vi "Write Setpoint.vi"(8 "error in (no error)":errorcluster, 10 "Setpoint":dbl=1.0, 11 "Percent Difference in":refnum<class "Percent Difference.lvclass">) -> (0 "error out":errorcluster, 3 "Percent Difference out":refnum<class "Percent Difference.lvclass">)   [LabVIEW 2021, in "Percent Difference.lvclass"]
uses:
  Percent Difference.lvclass
  Percent Difference.lvclass/Percent Difference.ctl
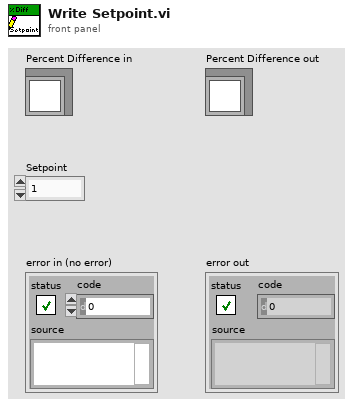
[diagram p1: front panel]
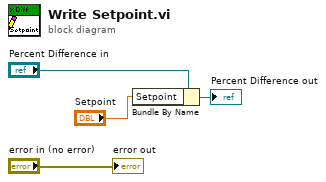
[diagram p0: block diagram]
diagram:
  n1 = Bundle By Name(cluster="Percent Difference in", "Setpoint"="Setpoint") -> (→"Percent Difference out":refnum<class "Percent Difference.lvclass">)
  "error out" <- "error in (no error)"
